vi "Start Root Controller.vi"() -> ()   [LabVIEW 2017, in "Controller Actor.lvlib" / "Controller.lvclass"]
uses:
  Controller.lvclass
  C:/Program Files (x86)/National Instruments/LabVIEW 2017/vi.lib/ActorFramework/Actor/Actor.lvclass
  Msmt Configuration/Controller Configuration.lvclass
  C:/Program Files (x86)/National Instruments/LabVIEW 2017/user.lib/Configuration Dialog Actor/Configuration.lvclass
  Msmt UI/Measurement UI.lvclass
  \\Mac\Home/Documents/MAL-Framework/user.lib/Common Components/User Interface/UI.lvclass
  <vilib>/ActorFramework/Actor/Actor.lvclass
panel:
  out "Path to config file":path
  out "error out":errorcluster
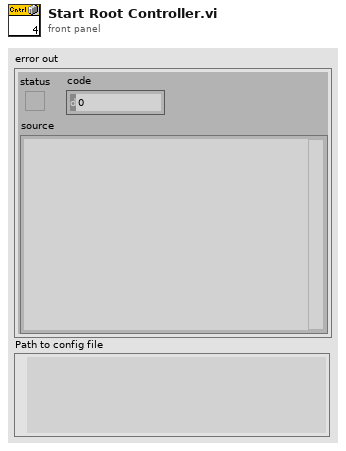
[diagram p1: front panel]
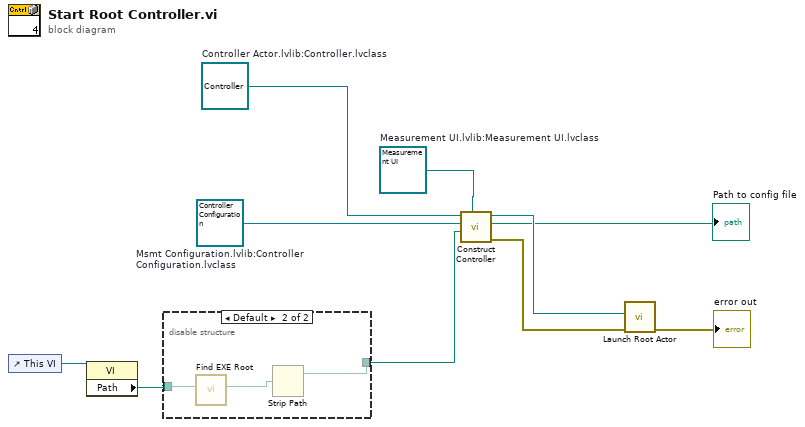
[diagram p0: block diagram]
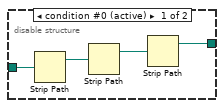
[diagram p2: hidden frame]
diagram:
  w2 = refnum<class "Measurement UI.lvclass"> refnum  # Measurement UI.lvlib:Measurement UI.lvclass
  w3 = refnum<class "Controller Configuration.lvclass"> refnum  # Msmt Configuration.lvlib:Controller Configuration.lvclass
  w10 = refnum<class "Controller.lvclass"> refnum  # Controller Actor.lvlib:Controller.lvclass
  n1 = control-ref of="This VI"() -> (w6:refnum<vi>)
  n2 = property class="VI"(reference=w6) -> ("Path"=w5:path)  [unwired: 1 in, 2 out]
  n3 = disable-structure shown="Default" {
    disable-tunnel: w5 -> [w13 w17]
    disable-tunnel: [w11 w15] -> w1
    frame condition #0 (active) {
      n4 = Strip Path(path=w13) -> (stripped path=w14:path)  [unwired: 1 out]
      n5 = Strip Path(path=w14) -> (stripped path=w12:path)  [unwired: 1 out]
      n6 = Strip Path(path=w12) -> (stripped path=w11:path)  [unwired: 1 out]
    }
    frame condition #1 {
      n7 = call "Find EXE Root.vi"("Path"=w17) -> ("Location of EXE"=w16:path)  [unwired: 10 in]
      n8 = Strip Path(path=w16) -> (stripped path=w15:path)  [unwired: 1 out]
    }
  }
  n9 = call "Construct Controller.vi"("UI.lvclass"=w2, "Root Path"=w1, "Configuration.lvlib:Configuration.lvclass"=w3, "Controller Actor.lvlib:Controller.lvclass"=w10) -> ("error out"=w8:errorcluster, "Path to config file"=→"Path to config file":path, "Controller Actor.lvlib:Controller.lvclass 2"=w9:refnum<class "Controller.lvclass">)  [unwired: 5 in]
  n10 = call <vilib>:"Launch Root Actor.vi"("error in (no error)"=w8, "Actor"=w9) -> ("error out"=→"error out":errorcluster)  [unwired: 8 in, 1 out]
